vi "Exercises_2-1.vi"() -> ()   [LabVIEW 2014]
panel:
  in  "Boolean":bool
  out "Seconds":dbl
  out "Minutes":dbl
  out "Hours":dbl
  in  "Total time in seconds":dbl
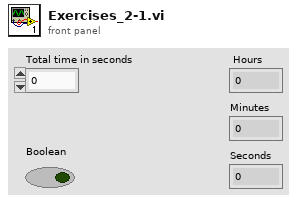
[diagram p1: front panel]
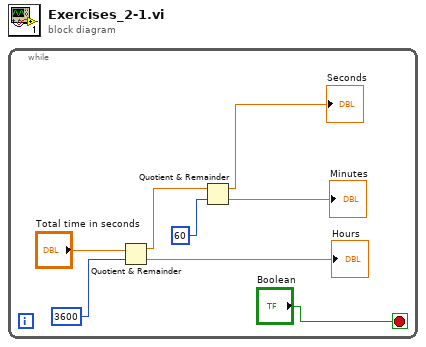
[diagram p0: block diagram]
diagram:
  n1 = while {
    stop <- "Boolean" stop-if-true
    n2 = Quotient & Remainder(x="Total time in seconds", y=3600) -> (x-y*floor(x/y)=w5:dbl, floor(x/y)=→"Hours":dbl)
    n3 = Quotient & Remainder(x=w5, y=60) -> (x-y*floor(x/y)=→"Seconds":dbl, floor(x/y)=→"Minutes":dbl)
  }
